vi "AVS_Done.vi"() -> (17 "Output Value":i32)   [LabVIEW 2016]
uses:
  Downloads/LinuxAPIselected/RedHat/libavs.so
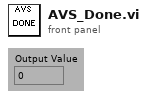
[diagram p1: front panel]
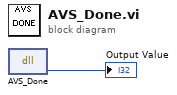
[diagram p0: block diagram]
diagram:
  n1 = dll-call lib="home/harini/Downloads/LinuxAPIselected/RedHat/libavs.so" fn="AVS_Done"() -> ("return type"=→"Output Value":i32)  [unwired: 3 in, 2 out]
